vi "Get HTTP Session Attributes.vi"(8 "error in (no error)":errorcluster, 11 "Web Request in":refnum<class "Web Request.lvclass">) -> (0 "error out":errorcluster, 2 "Username":string, 3 "Web Request out":refnum<class "Web Request.lvclass">)   [LabVIEW 2016, in "WSsupport.lvlib"]
uses:
  WSsupport.lvlib
  <vilib>/wsapi/Web Request.lvclass
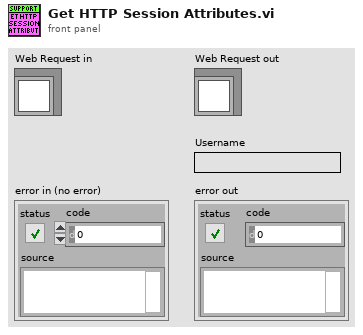
[diagram p1: front panel]
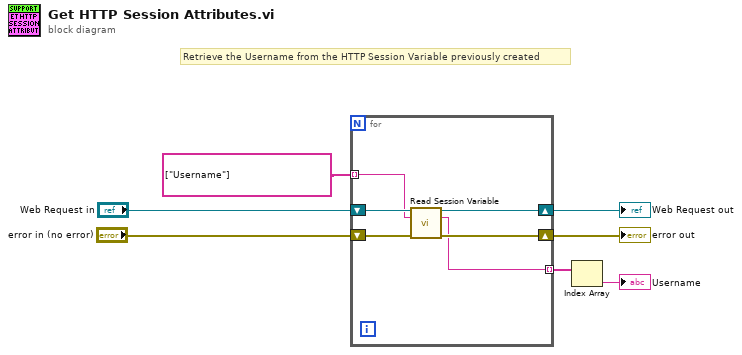
[diagram p0: block diagram]
diagram:
  # "Retrieve the Username from the HTTP Session Variable previously created"
  n1 = for {
    shift-right: [w12] -> w6
    shift-left: "Web Request in" -> [w11]
    shift-right: [w13] -> w7
    shift-left: "error in (no error)" -> [w10]
    tunnel: string[] ["Username"] -> [w9] mode=indexing
    tunnel: [w8] -> w2 mode=indexing
    n2 = call <vilib>:"Read Session Variable.vi"("LabVIEW Web Service Request"=w11, "key"=w9, "error in (no error)"=w10) -> ("LabVIEW Web Service Request out"=w12:refnum<class "Web Request.lvclass">, "value"=w8:string, "error out"=w13:errorcluster)  [unwired: 10 in]
  }
  "error out" <- w7
  "Web Request out" <- w6
  n3 = Index Array(array=w2) -> (element=→"Username":string)  [unwired: 1 in]
